vi "OE2011&OE2021_Configure Auto Chout Offest.vi"(7 "OE2011&OE2021_\nAuto Setting":cluster{"Auto CH Offest":bool, "CH Output":u16} {"CH Output" items=["CH1"=1, "CH2"=2]}, 8 "Error in (no error)":errorcluster caption="error out（no error）", 9 "Remote Mode":u16(ring) items=["USB", "RS232", "GPIB", "Ethernet"], 10 "Connection ID in":refnum<k5>, 11 "VISA resource name":refnum<visa-resource-name>) -> (0 "Error out":errorcluster caption="error out", 1 "Output String":string, 2 "Connection ID out":refnum<k5>, 3 "VISA resource  out":refnum<visa-resource-name>)   [LabVIEW 2011]
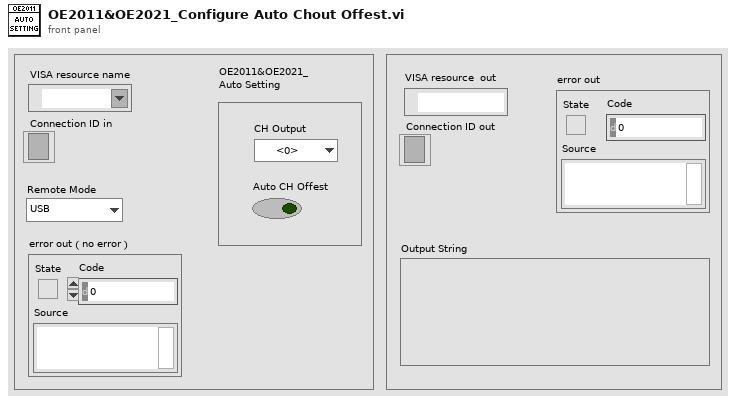
[diagram p1: front panel]
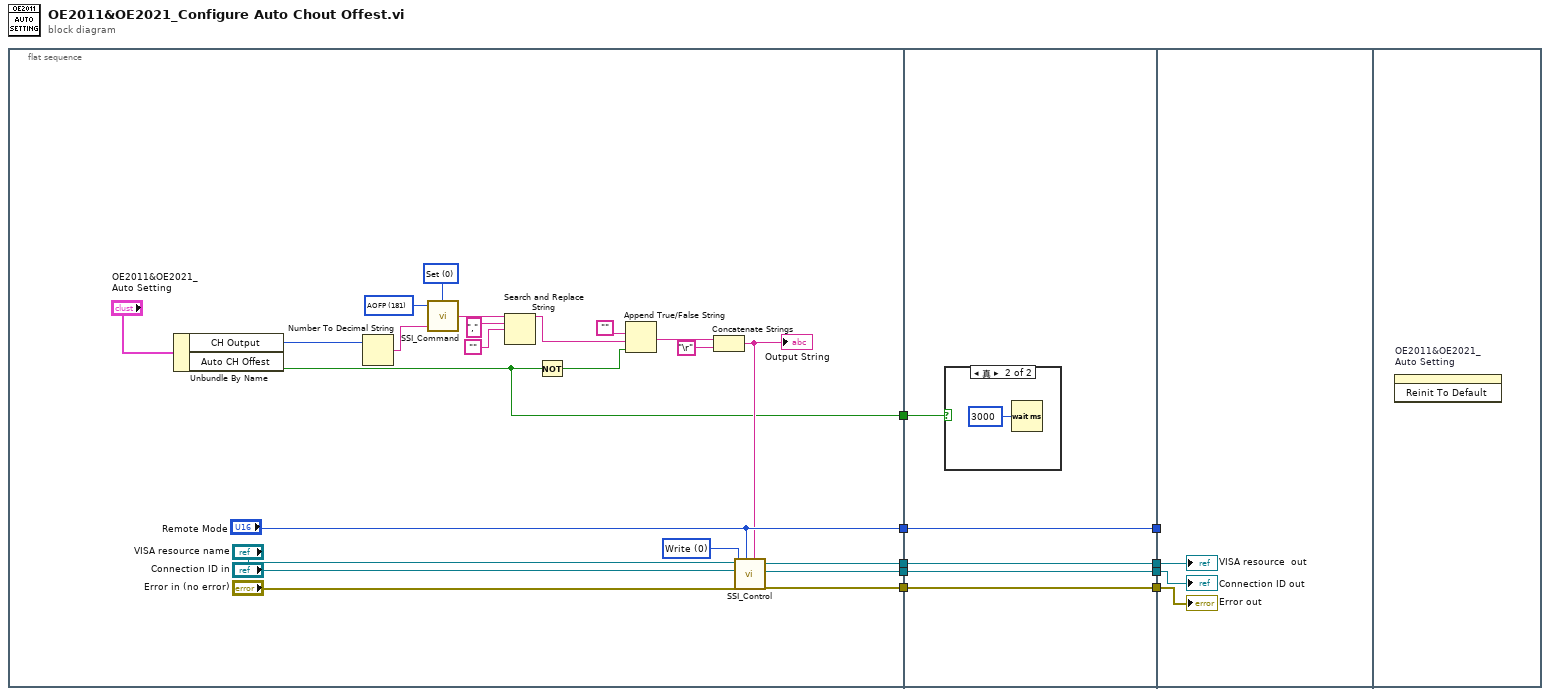
[diagram p0: block diagram]
diagram:
  n1 = flat-sequence {
    tunnel: [w28] -> w9
    tunnel: [w27] -> w8
    tunnel: [w26] -> w7
    tunnel: ["Remote Mode"] -> w3
    tunnel: [w11] -> w1
    tunnel: w9 -> [w37]
    tunnel: w8 -> [w36]
    tunnel: w7 -> [w35]
    tunnel: [w37] -> w6
    tunnel: [w36] -> w5
    tunnel: [w35] -> w4
    tunnel: w3 -> [w34]
    tunnel: [w34] -> w2
    tunnel: w1 -> [w33]
    tunnel: w6 -> [w40]
    tunnel: w5 -> [w41]
    tunnel: w4 -> [w39]
    tunnel: w2 -> [_]
    frame #0 {
      w19 = u16 181 items=["ISRC", "IGND", "ICPL", "ILIN", "PHAS", "FMOD", "RSLP", "FREQ", "SWPT", "SLLM", "SULM", "SSLL", "SSLG", "STLM", "SWRM", "IRNG", "SENS", "RMOD", "OFLT", "OFSL", "SYNC", "DMOD", "HARM", "DARB", "SWVT", "SLVL", "SVLL", "SVUL", "SVSL", "SVSG", "SVTM", "SVRM", "RALL", "SNAP", "OUTP", "OAUX", "COUT", "CAUX", "COFP", "CEXP", "FPOP", "OEXP", "*IDN", "*RST", "OVLD", "INOV", "GNOV", "*PLL", "SSET", "RSET", "AGAN", "APHS", "ARSV", "ASCL", "EQCD", "EQCS", "SPED", "SRAT", "SLEN", "SSLE", "STRG", "SPRM", "STRD", "PAUS", "REST", "SPTS", "TRCA", "TEMP", "RSTU", "INHZ", "DEQU", "SADD", "ARNG", "CSPE", "ISRCD", "IGNDD", "ICPLD", "ILIND", "PHASD", "FMODD", "RSLPD", "FREQD", "SWPTD", "SLLMD", "SULMD", "SSLLD", "SSLGD", "STLMD", "SWRMD", "SENSD", "RMODD", "OFLTD", "OFSLD", "SYNCD", "HARMD", "EQCDD", "EQCSD", "SNAPD", "OUTPD", "SWVTD", "SLVLD", "SVLLD", "SVULD", "SVSLD", "SVSGD", "SVTMD", "SVRMD", "SVDCD", "ARSVD", "AGAND", "APHSD", "ASCLD", "FPOPD", "CAUXD", "OEXPD", "SPEDD", "SRATD", "SLEND", "SSLED", "STRGD", "SPRMD", "STRDD", "PAUSD", "RESTD", "SPTSD", "TRCAD", "*IDND", "*RSTD", "INOVD", "GNOVD", "*PLLD", "SSETD", "RSETD", "RALLD", "NIPA", "NSMA", "NGWA", "NMAC", "NMOD", "TRIG", "TRCB", "INHZD", "ISAMD", "IRAGD", "RRAGD", "SOFFD", "DMODD", "COUTD", "COFPD", "CEXPD", "ARNGD", "OAUXD", "TRIM", "SUITD", "SNHZD", "AOFSD", "RSRC", "FEXT", "FINT", "DSRC", "DARF", "DEAF", "DREF", "SSRC", "STTL", "SIGO", "SLVL", "SOFF", "SPHS", "TPHS", "SMOD", "MARF", "AMSR", "AMDP", "FMSR", "FMDV", "PMSR", "PMDV", "CHDC", "AUXV", "AFLT", "AOFP"] ("Command Type")
      w14 = u16 0 items=["Set", "Query"] ("Opera")
      w29 = u16 0 items=["Write", "Read"] ("Control")
      n2 = Unbundle By Name("OE2011&OE2021_\nAuto Setting") -> ("CH Output"=w12:u16, "Auto CH Offest"=w11:bool)
      n3 = Number To Decimal String(number=w12) -> (decimal integer string=w13:string)  [unwired: 1 in]
      n4 = call "SSI_Command.vi"("Opera"=w14, "Paramter"=w13, "Command Type"=w19) -> ("Output string"=w20:string)  [unwired: 1 in]
      n5 = Search and Replace String(input string=w20, search string="," ("搜索字符串"), replace string="") -> (result string=w10:string)  [unwired: 5 in, 3 out]
      n6 = Not(x=w11) -> (.not. x?=w15:bool)
      n7 = Append True/False String(1:w15, 2:w10, 3:"") -> (0:w16:string)  [unwired: 1 in]
      n8 = Concatenate Strings(w16, "\r") -> (w17:string)
      "Output String" <- w17
      n9 = call "SSI_Control.vi"("Write Buffer"=w17, "Remote Mode"="Remote Mode", "Error in (no error)"="Error in (no error)", "Control"=w29, "Connection ID in"="Connection ID in", "VISA resource name"="VISA resource name") -> ("Error out"=w26:errorcluster, "Connection ID out"=w28:refnum<k5>, "VISA resource  out"=w27:refnum<visa-resource-name>)  [unwired: 2 in, 1 out]
    }
    frame #1 {
      n10 = case shown="真" w33 {
        frame False {
        }
        frame True {
          n11 = Wait (ms)(milliseconds to wait=u32 3000 ("等待时间（毫秒）")) -> ()  [unwired: 1 out]
        }
      }
    }
    frame #2 {
      "Error out" <- w39
      "Connection ID out" <- w40
      "VISA resource  out" <- w41
    }
    frame #3 {
      n12 = invoke on="OE2011&OE2021_\nAuto Setting" class="Clust (严格)" method="Reinit To Default"() -> ()  [unwired: 3 in, 3 out]
    }
  }
